vi "Launcher.vi"() -> (0 "error out":errorcluster)   [LabVIEW 2014]
uses:
  Camera Tester.lvclass
  <vilib>/ActorFramework/Actor/Actor.lvclass
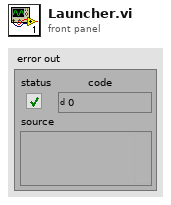
[diagram p1: front panel]
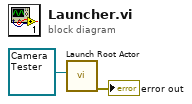
[diagram p0: block diagram]
diagram:
  n1 = call <vilib>:"Launch Root Actor.vi"("Actor"=refnum<class "Camera Tester.lvclass"> refnum ("Camera Tester.lvlib:Camera Tester.lvclass")) -> ("error out"=→"error out":errorcluster)  [unwired: 9 in, 1 out]
